vi "EZ Voltage.vi"(6 "AC/DC (F:DC)":bool, 7 "Scan List (empty)":string, 8 "error in (no error)":errorcluster, 9 "Range (5:Auto)":T2(ring)=enum."Auto", 10 "Resolution (5:Default)":T1(ring)=enum."Default", 11 "VISA Resource Name":refnum<visa-resource-name>="GPIB0::9::INSTR") -> (0 "error out":errorcluster, 2 "Output Array":dbl[](array[numeric]) format="%.2f", 3 "VISA Resource Name Out":refnum<visa-resource-name>)   [LabVIEW 2016, in "Agilent 34970.lvlib"]
doc: "This VI allows you to take simple voltage measurements from the instrument."
uses:
  Agilent 34970.lvlib
panel:
  out "read buffer":string
  out "concatenated string":string
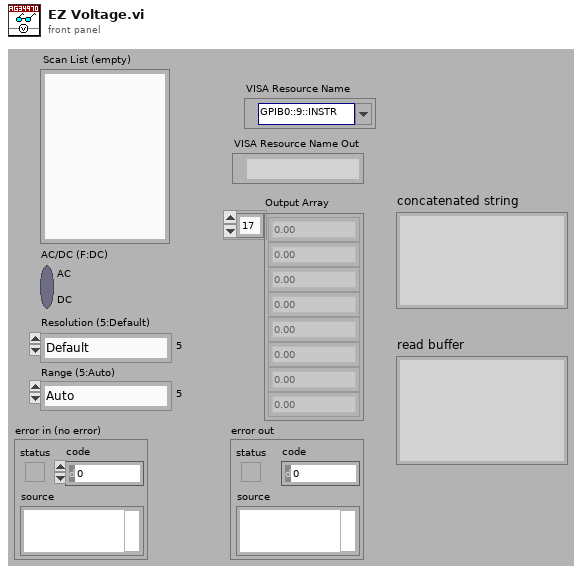
[diagram p1: front panel]
types:
  T1 = enum16{"4 1/2", "5 1/2", "6 1/2", "Least", "Highest", "Default"}
  T2 = enum16{"100 mV", "1 V", "10 V", "100 V", "300 V", "Auto", "Minimum", "Maximum"}
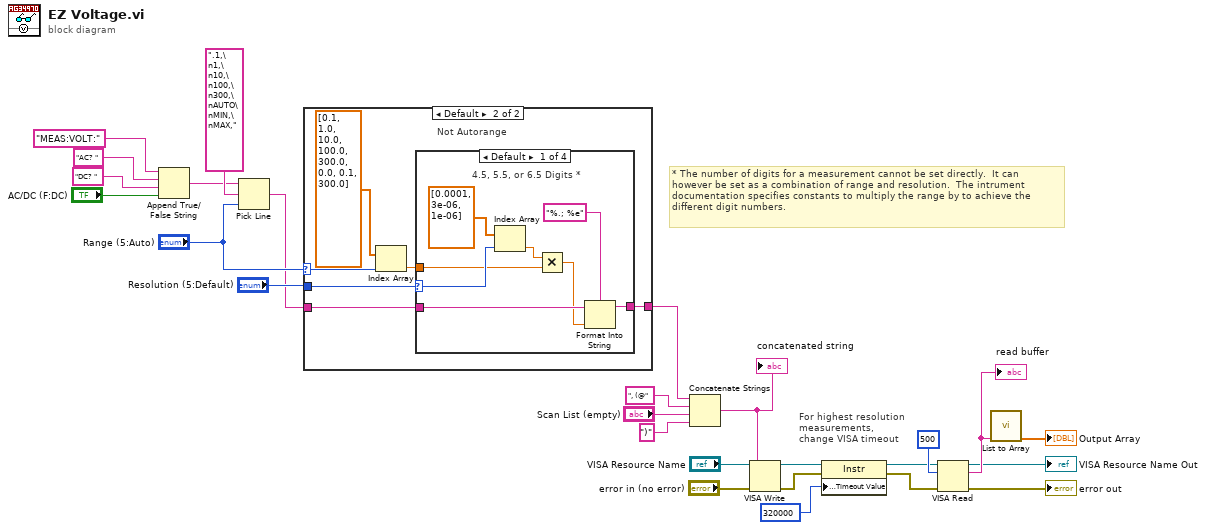
[diagram p0: block diagram]
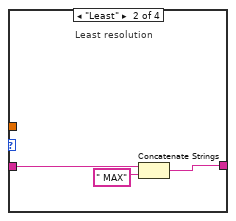
[diagram p3: hidden frame]
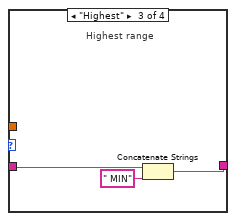
[diagram p4: hidden frame]
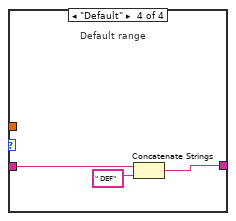
[diagram p5: hidden frame]
diagram:
  # "* The number of digits for a measurement cannot be set directly.  It can\nhowever be set as a combination of range and resolution.  The intrument\ndocumentation specifies constants to multiply the range by to achieve the\ndifferent digit numbers."
  # "For highest resolution\nmeasurements, \nchange VISA timeout"
  n1 = Append True/False String(1:"AC/DC (F:DC)", 2:"DC? ", 3:"AC? ", 4:"MEAS:VOLT:") -> (0:w5:string)
  n2 = Pick Line(string ("")=w5, multi-line string=".1,\n1,\n10,\n100,\n300,\nAUTO\nMIN,\nMAX,", line index="Range (5:Auto)") -> (output string=w2:string)
  n3 = case shown="Default" "Range (5:Auto)" {
    selector: "Range (5:Auto)" -> [_ w33]
    tunnel: [w27 w30] -> w1
    tunnel: w2 -> [w27 w29]
    tunnel: "Resolution (5:Default)" -> [_ w31]
    frame "Auto" {
      # "Autorange"
    }
    frame Default {
      # "Not Autorange"
      n4 = Index Array(array=dbl[] [0.1, 1.0, 10.0, 100.0, 300.0, 0.0, 0.1, 300.0], index=w33) -> (element=w28:dbl)
      n5 = case shown="Default" w31 {
        selector: w31 -> [w40 _ _ _]
        tunnel: [w34 w44 w47 w48] -> w30
        tunnel: w29 -> [w37 w43 w45 w49]
        tunnel: w28 -> [w39 _ _ _]
        frame Default {
          # "4.5, 5.5, or 6.5 Digits *"
          n6 = Index Array(array=dbl[] [0.0001, 3e-06, 1e-06], index=w40) -> (element=w38:dbl)
          n7 = Multiply(x=w38, y=w39) -> (x*y=w36:dbl)
          n8 = Format Into String(format string="%.; %e", initial string=w37, w36) -> (resulting string=w34:string)  [unwired: 1 in, 1 out]
        }
        frame "Least" {
          # "Least resolution"
          n9 = Concatenate Strings(w43, " MAX" ("string")) -> (w44:string)
        }
        frame "Highest" {
          # "Highest range"
          n10 = Concatenate Strings(w45, " MIN" ("string")) -> (w47:string)
        }
        frame "Default" {
          # "Default range"
          n11 = Concatenate Strings(w49, " DEF" ("string")) -> (w48:string)
        }
      }
    }
  }
  n12 = Concatenate Strings(w1, ", (@", "Scan List (empty)", ")") -> (w13:string)
  "concatenated string" <- w13
  n13 = VISA Write(VISA resource name="VISA Resource Name", write buffer=w13, error in (no error)="error in (no error)") -> (VISA resource name out=w23:refnum<visa-resource-name>, error out=w22:errorcluster)  [unwired: 1 out]
  n14 = property class="Instr"(reference=w23, error in=w22, "General Settings:Timeout Value"=u32 320000 ("Tmo Value")) -> (reference out=w20:refnum<visa-resource-name>, error out=w21:errorcluster)
  n15 = VISA Read(VISA resource name=w20, byte count=u32 500 ("byte count (0)"), error in (no error)=w21) -> (VISA resource name out=→"VISA Resource Name Out":refnum<visa-resource-name>, read buffer=w14:string, error out=→"error out":errorcluster)  [unwired: 1 out]
  "read buffer" <- w14
  n16 = call "List to Array.vi"("List (empty)"=w14) -> ("Output Number Array"=→"Output Array":dbl[])  [unwired: 9 in, 1 out]
